vi "select ROIS.vi"(8 "error in (no error)":errorcluster, 11 "Cascade in":refnum<class "Cascade.lvclass">) -> (0 "error out":errorcluster, 3 "Cascade out":refnum<class "Cascade.lvclass">)   [LabVIEW 2012, in "Cascade.lvclass"]
uses:
  Cascade.lvclass
  Cascade.lvclass/Cascade.ctl
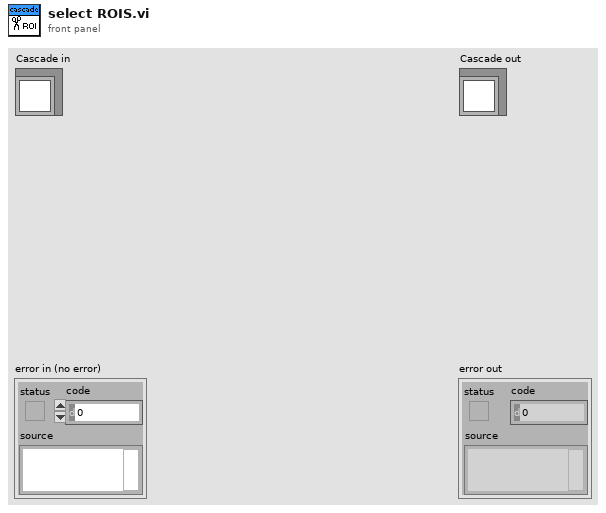
[diagram p1: front panel]
types:
  T1 = typedef "IMAQ Rectangle" = cluster{"Left":i32, "Top":i32, "Right":i32, "Bottom":i32, "Rotation":dbl}
  T2 = typedef "IMAQ Image.ctl" = refnum<image>
  T3 = typedef "ROI Descriptor" = cluster{"Global Rectangle":i32[], "Contours":cluster{"ID":enum32{"External", "Internal"}, "Type":u32, "Coordinates":i32[]}[]}
  T4 = cluster{"[0]":i32, "[1]":i32, "[2]":i32, "[3]":i32, "[4]":i32, "[5]":i32, "[6]":i32, "[7]":i32, "[8]":i32}
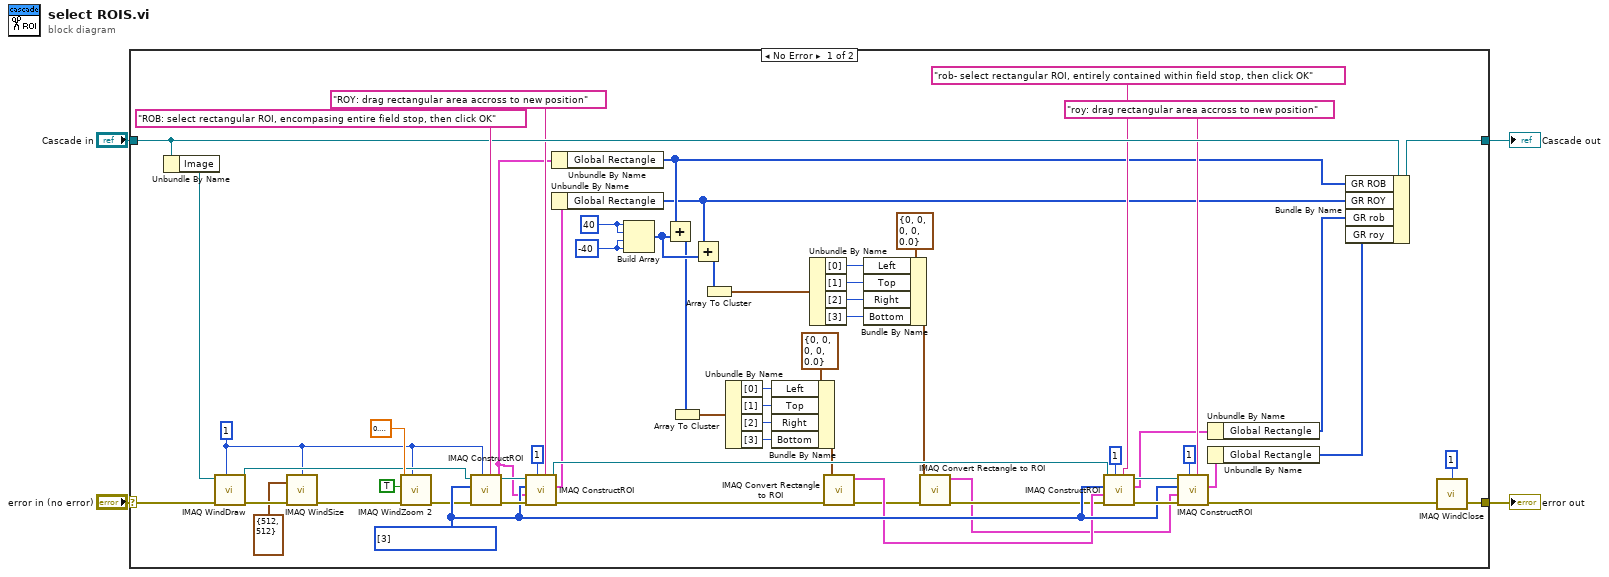
[diagram p0: block diagram]
diagram:
  n1 = case shown="No Error" "error in (no error)" {
    selector: "error in (no error)" -> [w60 w66]
    tunnel: [w47 w66] -> w3
    tunnel: [w44 w65] -> w1
    tunnel: "Cascade in" -> [w45 w65]
    frame No Error {
      w31 = -40
      w32 = 40
      w34 = 1 ("Window Number (0...15)")
      w50 = u32[] [3] items=["No Selection", "Point", "Line", "Rectangle", "Oval", "Polygon", "Freehand Region", "Annulus", "Zoom", "Pan", "Broken Line", "Freehand Line", "Rotated Rectangle"] ("Tools")
      n2 = Unbundle By Name(w45) -> ("Image"=w61:T2)
      n3 = call "IMAQ WindDraw"("Window Number (0...15)"=w34, "error in (no error)"=w60, "Image"=w61) -> ("error out"=w36:errorcluster, "Image Out (duplicate)"=w63:T2)  [unwired: 7 in]
      n4 = call "IMAQ WindSize"("error in (no error)"=w36, "Width & Height"=cluster{"Width":i32, "Height":i32} {"Width"=512, "Height"=512}, "Window Number"=w34) -> ("error out"=w35:errorcluster)  [unwired: 3 in, 2 out]
      n5 = call "IMAQ WindZoom 2"("Window Number (0...15)"=w34, "error in (no error)"=w35, "Zoom to Fit? (False)"=TRUE, "Zoom Factor"=sgl 0.9) -> ("error out"=w37:errorcluster)  [unwired: 4 in, 3 out]
      n6 = call "IMAQ ConstructROI"("Prompt"="ROB: select rectangular ROI, encompasing entire field stop, then click OK", "Window Number (-1...15)"=w34, "error in (no error)"=w37, "Tools"=w50, "Image"=w63) -> ("error out"=w57:errorcluster, "ROI Descriptor Out"=w27:T3, "Image Out (duplicate)"=w56:T2)  [unwired: 3 in, 1 out]
      n7 = call "IMAQ ConstructROI"("Prompt"="ROY: drag rectangular area accross to new position", "Window Number (-1...15)"=1, "error in (no error)"=w57, "ROI Descriptor In (None)"=w27, "Tools"=w50, "Image"=w56) -> ("error out"=w15:errorcluster, "ROI Descriptor Out"=w26:T3, "Image Out (duplicate)"=w52:T2)  [unwired: 2 in, 1 out]
      n8 = Unbundle By Name(w27) -> ("Global Rectangle"=w30:i32[])
      n9 = Unbundle By Name(w26) -> ("Global Rectangle"=w29:i32[])
      n10 = Build Array(w32, w32, w31, w31) -> (w28:i32[])
      n11 = Add(x=w30, y=w28) -> (x+y=w24:i32[])
      n12 = Array To Cluster(array=w24) -> (cluster=w23:T4)
      n13 = Add(x=w29, y=w28) -> (x+y=w12:i32[])
      n14 = Array To Cluster(array=w12) -> (cluster=w11:T4)
      n15 = Unbundle By Name(w23) -> ("[0]"=w22:i32, "[1]"=w21:i32, "[2]"=w20:i32, "[3]"=w19:i32)
      n16 = Bundle By Name(cluster=T1 {"Left"=0, "Top"=0, "Right"=0, "Bottom"=0, "Rotation"=0.0} ("Rectangle"), "Left"=w22, "Top"=w21, "Right"=w20, "Bottom"=w19) -> (w18:T1)
      n17 = Unbundle By Name(w11) -> ("[0]"=w10:i32, "[1]"=w9:i32, "[2]"=w8:i32, "[3]"=w7:i32)
      n18 = call "IMAQ Convert Rectangle to ROI"("error in (no error)"=w15, "Rectangle"=w18) -> ("error out"=w16:errorcluster, "ROI Descriptor"=w17:T3)  [unwired: 7 in]
      n19 = Bundle By Name(cluster=T1 {"Left"=0, "Top"=0, "Right"=0, "Bottom"=0, "Rotation"=0.0} ("Rectangle"), "Left"=w10, "Top"=w9, "Right"=w8, "Bottom"=w7) -> (w6:T1)
      n20 = call "IMAQ Convert Rectangle to ROI"("error in (no error)"=w16, "Rectangle"=w6) -> ("error out"=w14:errorcluster, "ROI Descriptor"=w5:T3)  [unwired: 7 in]
      n21 = call "IMAQ ConstructROI"("Prompt"="rob- select rectangular ROI, entirely contained within field stop, then click OK", "Window Number (-1...15)"=1, "error in (no error)"=w14, "ROI Descriptor In (None)"=w17, "Tools"=w50, "Image"=w52) -> ("error out"=w53:errorcluster, "ROI Descriptor Out"=w38:T3, "Image Out (duplicate)"=w51:T2)  [unwired: 2 in, 1 out]
      n22 = call "IMAQ ConstructROI"("Prompt"="roy: drag rectangular area accross to new position", "Window Number (-1...15)"=1, "error in (no error)"=w53, "ROI Descriptor In (None)"=w5, "Tools"=w50, "Image"=w51) -> ("error out"=w46:errorcluster, "ROI Descriptor Out"=w49:T3)  [unwired: 2 in, 2 out]
      n23 = Unbundle By Name(w38) -> ("Global Rectangle"=w43:i32[])
      n24 = Unbundle By Name(w49) -> ("Global Rectangle"=w42:i32[])
      n25 = Bundle By Name(cluster=w45, "GR ROB"=w30, "GR ROY"=w29, "GR rob"=w43, "GR roy"=w42) -> (w44:refnum<class "Cascade.lvclass">)
      n26 = call "IMAQ WindClose"("Window Number (0...15)"=1, "error in (no error)"=w46) -> ("error out"=w47:errorcluster)  [unwired: 4 in]
    }
    frame Error {
    }
  }
  "error out" <- w3
  "Cascade out" <- w1
